vi "read frame string.vi"(8 "error in":errorcluster, 10 "frame number":u32, 11 "file string":string) -> (0 "error out":errorcluster, 2 "found":bool, 3 "<f> string":string, 4 "<f> end pos":i32)   [LabVIEW 2018, in "Frame Analizer.lvclass"]
uses:
  Frame Analizer.lvclass
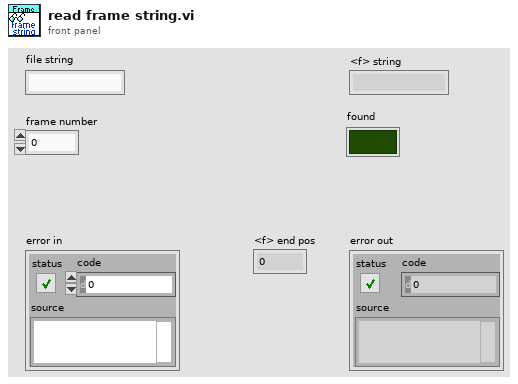
[diagram p1: front panel]
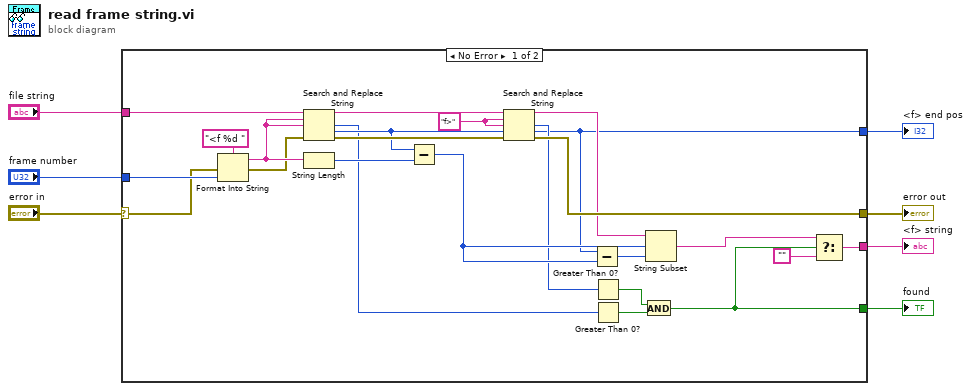
[diagram p0: block diagram]
diagram:
  n1 = case shown="No Error" "error in" {
    selector: "error in" -> [w26 w32]
    tunnel: "file string" -> [w30 _]
    tunnel: "frame number" -> [w29 _]
    tunnel: [w28 w32] -> w5
    tunnel: [w14 _] -> w4
    tunnel: [w9 _] -> w2
    tunnel: [w8 _] -> w1
    frame No Error {
      w20 = "f>" ("format string")
      n2 = Format Into String(format string="<f %d ", error in=w26, w29) -> (resulting string=w27:string, error out=w17:errorcluster)  [unwired: 1 in]
      n3 = Search and Replace String(input string=w30, search string=w27, replace string=w27, error in=w17) -> (result string=w25:string, number of replacements=w16:i32, offset past replacement=w22:i32, error out=w24:errorcluster)  [unwired: 4 in]
      n4 = String Length(string=w27) -> (length=w21:i32)
      n5 = Subtract(x=w22, y=w21) -> (x-y=w19:i32)
      n6 = Search and Replace String(input string=w25, search string=w20, replace string=w20, offset=w22, error in=w24) -> (result string=w23:string, number of replacements=w12:i32, offset past replacement=w8:i32, error out=w28:errorcluster)  [unwired: 3 in]
      n7 = Subtract(x=w8, y=w19) -> (x-y=w18:i32)
      n8 = Greater Than 0?(x=w12) -> (x > 0?=w11:bool)
      n9 = Greater Than 0?(x=w16) -> (x > 0?=w10:bool)
      n10 = And(x=w11, y=w10) -> (x .and. y?=w9:bool)
      n11 = String Subset(string=w23, offset (0)=w19, length (rest)=w18) -> (substring=w13:string)
      n12 = Select(t=w13, s=w9, f="") -> (s? t:f=w14:string)
    }
    frame Error {
    }
  }
  "error out" <- w5
  "<f> string" <- w4
  "found" <- w2
  "<f> end pos" <- w1
